vi "solar_cfg Core Edit.vi"(6 "Write Comments? (T)":bool=TRUE, 7 "Action (Read)":enum8{"Read", "Write", "Parse", "Build"}(ring), 8 "error in (no error)":errorcluster, 9 "kvc in":string[](array[string]), 10 "Section/String in":string, 11 "Sections in":cluster{"Section":string, "kvc":string[][]}[](array[cluster])) -> (0 "error out":errorcluster, 1 "Found?":bool, 2 "Value/String out":string, 3 "Sections out":cluster{"Section":string, "kvc":string[][]}[](array[cluster]), 5 "Dirty?":bool)   [LabVIEW 2018]
doc: "This VI parses the configuration string to sections, keys, values and comments."
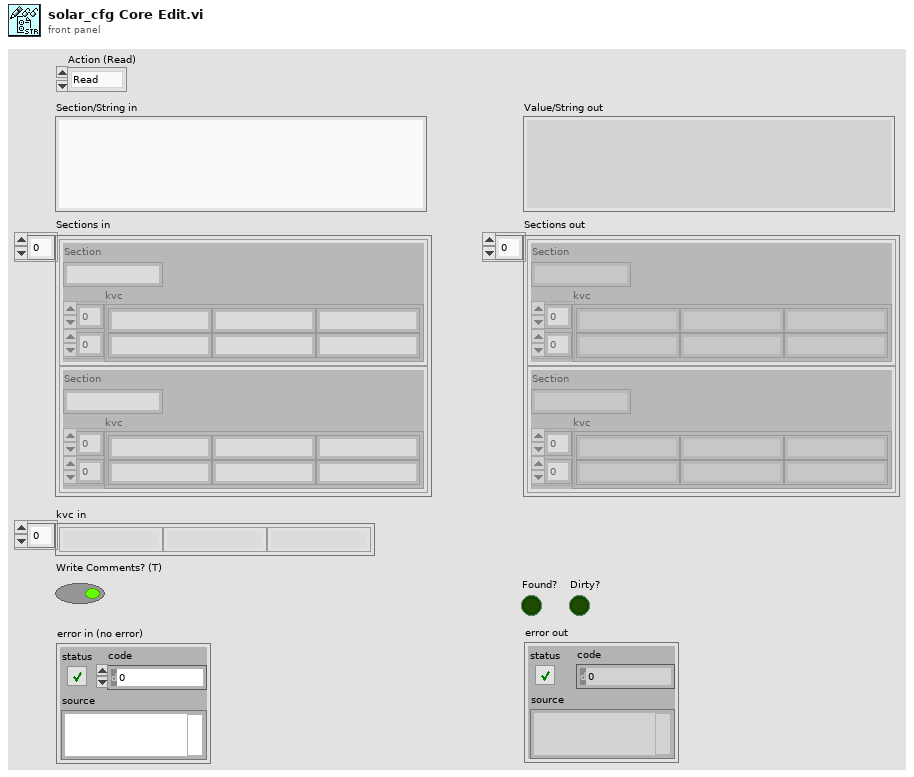
[diagram p1: front panel]
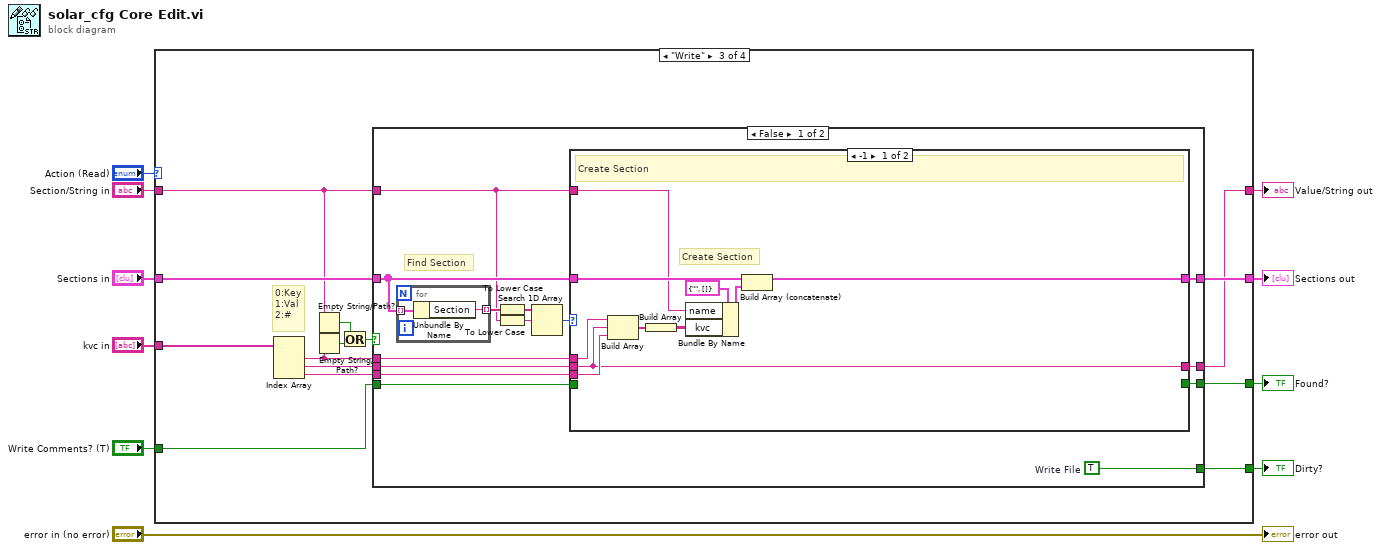
[diagram p0: block diagram]
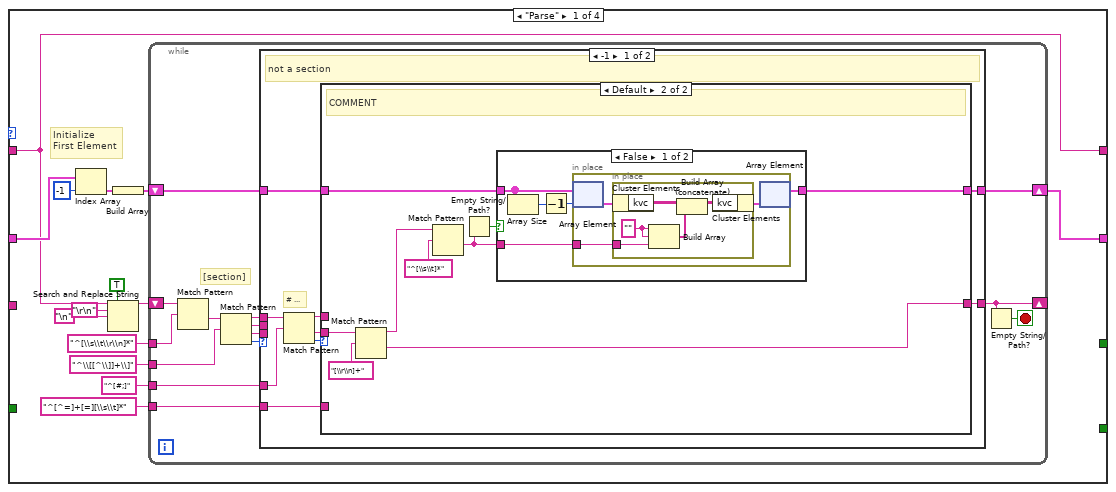
[diagram p2: hidden frame]
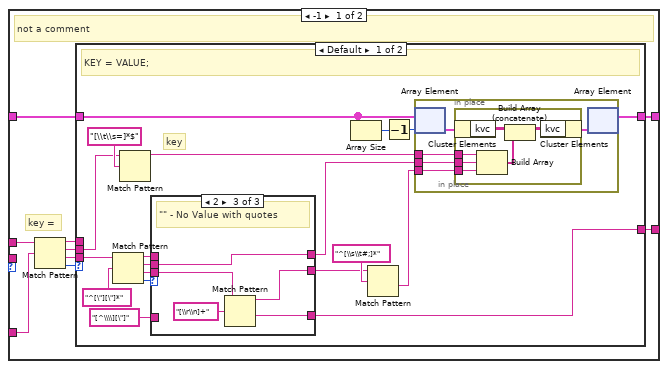
[diagram p3: hidden frame]
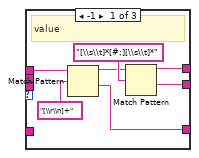
[diagram p4: hidden frame]
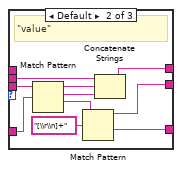
[diagram p5: hidden frame]
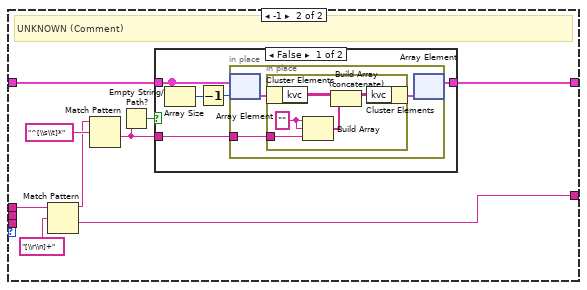
[diagram p6: hidden frame]
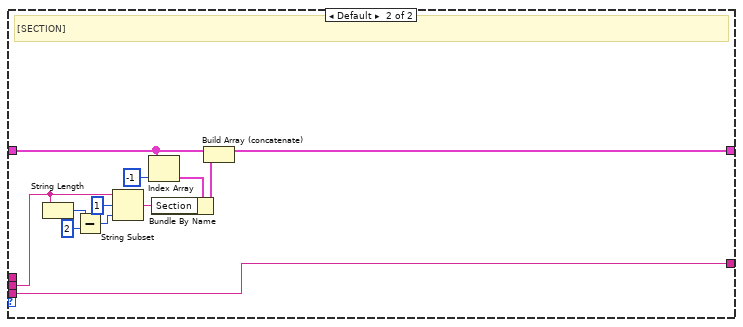
[diagram p9: hidden frame]
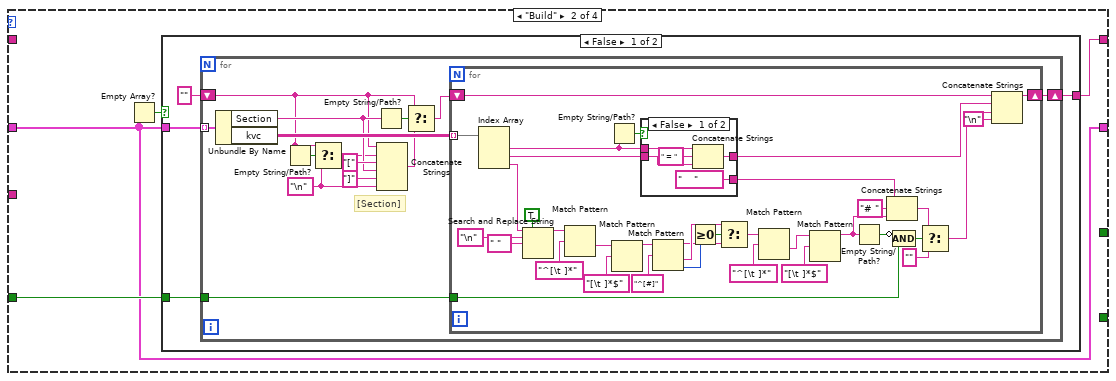
[diagram p10: hidden frame]
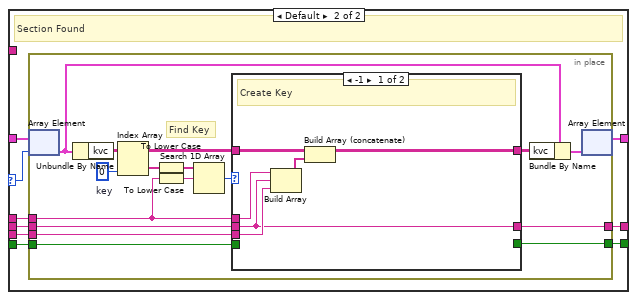
[diagram p13: hidden frame]
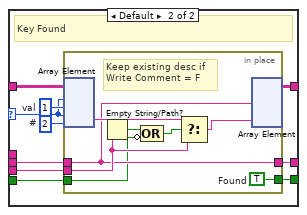
[diagram p14: hidden frame]
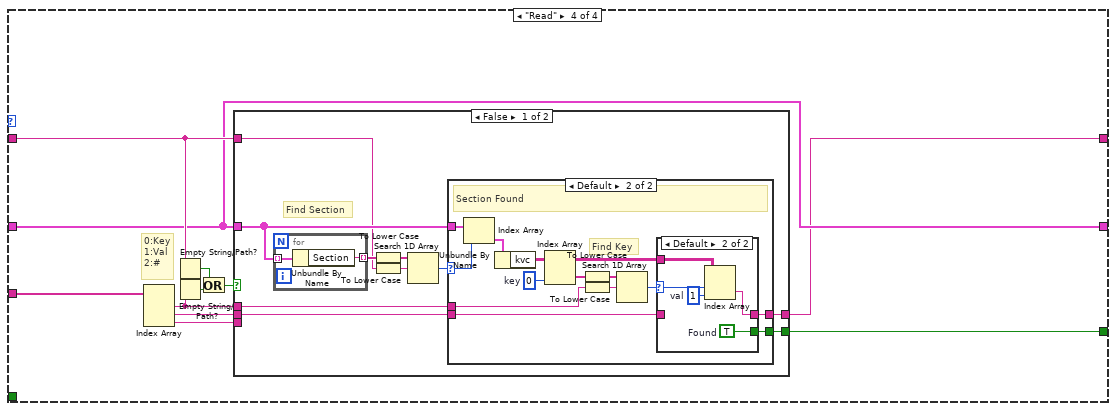
[diagram p16: hidden frame]
diagram:
  n1 = case shown="\"Write\"" "Action (Read)" {
    tunnel: "Section/String in" -> [w12 _ w233 w328]
    tunnel: [w11 w168 w241 w320] -> w9
    tunnel: [w12 w170 w232 w319] -> w7
    tunnel: "Sections in" -> [w13 w168 w242 w320]
    tunnel: "Write Comments? (T)" -> [_ w169 w231 _]
    tunnel: "kvc in" -> [_ _ w240 w329]
    tunnel: [_ _ w239 w327] -> w3
    tunnel: [_ _ w238 _] -> w2
    frame "Parse" {
      # "Initialize\nFirst Element"
      n2 = Index Array(array=w13, index=-1) -> (element=w19:cluster{"Section":string, "kvc":string[][]})
      n3 = Search and Replace String(replace all?=TRUE ("replace all? (F)"), input string=w12, search string="\r\n" ("End of Line Constant"), replace string="\n" ("Line Feed Constant")) -> (result string=w24:string)  [unwired: 4 in, 3 out]
      n4 = Build Array(w19) -> (w18:cluster{"Section":string, "kvc":string[][]}[])
      n5 = while {
        shift-right: [w30] -> _
        shift-left: w24 -> [w38]
        shift-right: [w31] -> w11
        shift-left: w18 -> [w32]
        tunnel: "^[\\s\\t\\r\\n]*" ("regular expression") -> [w28]
        tunnel: "^\\[[^\\]]+\\]" -> [w27]
        tunnel: "^[#;]" -> [w26]
        tunnel: "^[^=]+[=][\\s\\t]*" -> [w25]
        stop <- w29 stop-if-true
        # "[section]"
        n6 = Match Pattern(string=w38, regular expression=w28) -> (after substring=w37:string)  [unwired: 1 in, 3 out]
        n7 = Match Pattern(string=w37, regular expression=w27) -> (before substring=w35:string, match substring=w34:string, after substring=w33:string, offset past match=w36:i32)  [unwired: 1 in]
        n8 = case shown="-1" w36 {
          tunnel: w35 -> [w47 _]
          tunnel: w34 -> [_ w164]
          tunnel: w33 -> [_ w166]
          tunnel: [w42 w166] -> w30
          tunnel: w32 -> [w44 w159]
          tunnel: [w45 w160] -> w31
          tunnel: w26 -> [w40 _]
          tunnel: w25 -> [w39 _]
          frame -1 {
            # "# ..."
            # "not a section"
            n9 = Match Pattern(string=w47, regular expression=w40) -> (before substring=w41:string, after substring=w43:string, offset past match=w46:i32)  [unwired: 1 in, 1 out]
            n10 = case shown="Default" w46 {
              tunnel: [w54 w139] -> w45
              tunnel: w44 -> [w53 w140]
              tunnel: w43 -> [_ w137]
              tunnel: [w49 w136] -> w42
              tunnel: w41 -> [w56 _]
              tunnel: w39 -> [w48 _]
              frame -1 {
                # "key ="
                # "not a comment"
                n11 = Match Pattern(string=w56, regular expression=w48) -> (before substring=w52:string, match substring=w50:string, after substring=w51:string, offset past match=w55:i32)  [unwired: 1 in]
                n12 = case shown="Default" w55 {
                  tunnel: [w72 w116] -> w54
                  tunnel: w53 -> [w73 w117]
                  tunnel: w52 -> [_ w114]
                  tunnel: w51 -> [w67 _]
                  tunnel: w50 -> [w70 _]
                  tunnel: [w58 w113] -> w49
                  frame Default {
                    # "key"
                    # "KEY = VALUE;"
                    n13 = Match Pattern(string=w67, regular expression="^[\"][\"]*") -> (before substring=w57:string, match substring=w61:string, after substring=w64:string, offset past match=w65:i32)  [unwired: 1 in]
                    n14 = Match Pattern(string=w70, regular expression="[\\t\\s=]*$") -> (before substring=w69:string)  [unwired: 1 in, 3 out]
                    n15 = case shown="2" w65 {
                      tunnel: w64 -> [_ w92 w94]
                      tunnel: "[^\\\\][\"]" -> [_ w91 _]
                      tunnel: [w77 w83 w93] -> w62
                      tunnel: w61 -> [_ w86 w93]
                      tunnel: [w76 w88 w96] -> w60
                      tunnel: [w80 w87 w95] -> w58
                      tunnel: w57 -> [w81 _ _]
                      frame -1 {
                        # "value"
                        n16 = Match Pattern(string=w81, regular expression="[\\r\\n]+") -> (before substring=w78:string, after substring=w80:string)  [unwired: 1 in, 2 out]
                        n17 = Match Pattern(string=w78, regular expression="[\\s\\t]*[#;][\\s\\t]*") -> (before substring=w77:string, after substring=w76:string)  [unwired: 1 in, 2 out]
                      }
                      frame Default {
                        # "\"value\""
                        n18 = Match Pattern(string=w92, regular expression=w91) -> (before substring=w85:string, match substring=w84:string, after substring=w89:string)  [unwired: 1 in, 1 out]
                        n19 = Match Pattern(string=w89, regular expression="[\\r\\n]+") -> (before substring=w88:string, after substring=w87:string)  [unwired: 1 in, 2 out]
                        n20 = Concatenate Strings(w86, w85, w84) -> (w83:string)
                      }
                      frame 2 {
                        # "\"\" - No Value with quotes"
                        n21 = Match Pattern(string=w94, regular expression="[\\r\\n]+") -> (before substring=w96:string, after substring=w95:string)  [unwired: 1 in, 2 out]
                      }
                    }
                    n22 = Array Size(array=w73) -> (size(s)=w75:i32)
                    n23 = Match Pattern(string=w60, regular expression="^[\\s\\t#;]*") -> (after substring=w59:string)  [unwired: 1 in, 3 out]
                    n24 = Decrement(x=w75) -> (x-1=w74:i32)
                    n25 = in-place {
                      in-place-border: w59 -> [w101]
                      in-place-border: w69 -> [w99]
                      in-place-border: w62 -> [w98]
                      n26 = in-place-array #1(w73, w74) -> (w102:cluster{"Section":string, "kvc":string[][]})
                      n27 = in-place {
                        in-place-border: w101 -> [w106]
                        in-place-border: w99 -> [w104]
                        in-place-border: w98 -> [w103]
                        n28 = in-place-cluster #2(w102) -> ("kvc"=w108:string[][])
                        n29 = Build Array(w104, w103, w106) -> (w105:string[])
                        n30 = Build Array (concatenate)(w108, w105) -> (w107:string[][])
                        n31 = in-place-cluster #2("kvc"=w107) -> (w100:cluster{"Section":string, "kvc":string[][]})
                      }
                      n32 = in-place-array #1(w100) -> (w72:cluster{"Section":string, "kvc":string[][]}[])  [unwired: 1 out]
                    }
                  }
                  frame -1 {
                    # "UNKNOWN (Comment)"
                    n33 = Match Pattern(string=w114, regular expression="[\\r\\n]+") -> (before substring=w110:string, after substring=w113:string)  [unwired: 1 in, 2 out]
                    n34 = Match Pattern(string=w110, regular expression="^[\\s\\t]*") -> (after substring=w109:string)  [unwired: 1 in, 3 out]
                    n35 = Empty String/Path?(string/path=w109) -> (empty?=w112:bool)
                    n36 = case shown="False" w112 {
                      tunnel: w117 -> [w120 w131]
                      tunnel: [w119 w131] -> w116
                      tunnel: w109 -> [w118 _]
                      frame False {
                        n37 = Array Size(array=w120) -> (size(s)=w122:i32)
                        n38 = Decrement(x=w122) -> (x-1=w121:i32)
                        n39 = in-place {
                          in-place-border: w118 -> [w124]
                          n40 = in-place-array #3(w120, w121) -> (w125:cluster{"Section":string, "kvc":string[][]})
                          n41 = in-place {
                            in-place-border: w124 -> [w127]
                            w128 = ""
                            n42 = in-place-cluster #4(w125) -> ("kvc"=w130:string[][])
                            n43 = Build Array(w128, w128, w127) -> (w126:string[])
                            n44 = Build Array (concatenate)(w130, w126) -> (w129:string[][])
                            n45 = in-place-cluster #4("kvc"=w129) -> (w123:cluster{"Section":string, "kvc":string[][]})
                          }
                          n46 = in-place-array #3(w123) -> (w119:cluster{"Section":string, "kvc":string[][]}[])  [unwired: 1 out]
                        }
                      }
                      frame True {
                      }
                    }
                  }
                }
              }
              frame Default {
                # "COMMENT"
                n47 = Match Pattern(string=w137, regular expression="[\\r\\n]+") -> (before substring=w132:string, after substring=w136:string)  [unwired: 1 in, 2 out]
                n48 = Match Pattern(string=w132, regular expression="^[\\s\\t]*") -> (after substring=w133:string)  [unwired: 1 in, 3 out]
                n49 = Empty String/Path?(string/path=w133) -> (empty?=w135:bool)
                n50 = case shown="False" w135 {
                  tunnel: w140 -> [w145 w154]
                  tunnel: [w142 w154] -> w139
                  tunnel: w133 -> [w141 _]
                  frame False {
                    n51 = Array Size(array=w145) -> (size(s)=w144:i32)
                    n52 = Decrement(x=w144) -> (x-1=w143:i32)
                    n53 = in-place {
                      in-place-border: w141 -> [w147]
                      n54 = in-place-array #5(w145, w143) -> (w148:cluster{"Section":string, "kvc":string[][]})
                      n55 = in-place {
                        in-place-border: w147 -> [w150]
                        w151 = ""
                        n56 = in-place-cluster #6(w148) -> ("kvc"=w153:string[][])
                        n57 = Build Array(w151, w151, w150) -> (w149:string[])
                        n58 = Build Array (concatenate)(w153, w149) -> (w152:string[][])
                        n59 = in-place-cluster #6("kvc"=w152) -> (w146:cluster{"Section":string, "kvc":string[][]})
                      }
                      n60 = in-place-array #5(w146) -> (w142:cluster{"Section":string, "kvc":string[][]}[])  [unwired: 1 out]
                    }
                  }
                  frame True {
                  }
                }
              }
            }
          }
          frame Default {
            # "[SECTION]"
            n61 = String Length(string=w164) -> (length=w163:i32)
            n62 = Subtract(x=w163, y=2) -> (x-y=w162:i32)
            n63 = String Subset(string=w164, offset (0)=1, length (rest)=w162) -> (substring=w156:string)
            n64 = Index Array(array=w159, index=-1) -> (element=w157:cluster{"Section":string, "kvc":string[][]})
            n65 = Bundle By Name(cluster=w157, "Section"=w156) -> (w155:cluster{"Section":string, "kvc":string[][]})
            n66 = Build Array (concatenate)(w159, w155) -> (w160:cluster{"Section":string, "kvc":string[][]}[])
          }
        }
        n67 = Empty String/Path?(string/path=w30) -> (empty?=w29:bool)
      }
    }
    frame "Build" {
      n68 = Empty Array?(array=w168) -> (empty?=w167:bool)
      n69 = case shown="False" w167 {
        tunnel: w168 -> [w173 _]
        tunnel: [w172 _] -> w170
        tunnel: w169 -> [w171 _]
        frame False {
          n70 = for {
            tunnel: w173 -> [w188] mode=indexing
            shift-right: [w187] -> w172
            shift-left: "" -> [w177]
            tunnel: w171 -> [w186]
            w175 = "\n" ("string")
            # "[Section]"
            n71 = Unbundle By Name(w188) -> ("Section"=w180:string, "kvc"=w185:string[][])
            n72 = Empty String/Path?(string/path=w177) -> (empty?=w178:bool)
            n73 = Select(t=w177, s=w178, f=w175) -> (s? t:f=w176:string)
            n74 = Empty String/Path?(string/path=w180) -> (empty?=w184:bool)
            n75 = Concatenate Strings(w177, w176, "[" ("string"), w180, "]" ("string"), w175) -> (w183:string)
            n76 = Select(t=w177, s=w184, f=w183) -> (s? t:f=w179:string)
            n77 = for {
              tunnel: w186 -> [w201]
              tunnel: w185 -> [w195] mode=indexing
              shift-right: [w221] -> w187
              shift-left: w179 -> [w218]
              n78 = Index Array(array=w195) -> (element #1=w220:string, element #2=w219:string, element #3=w215:string)  [unwired: 3 in]
              n79 = Search and Replace String(replace all?=TRUE ("replace all? (F)"), input string=w215, search string="\n", replace string=" " ("replace string (\"\")")) -> (result string=w214:string)  [unwired: 4 in, 3 out]
              n80 = Match Pattern(string=w214, regular expression="^[\t ]*") -> (after substring=w212:string)  [unwired: 1 in, 3 out]
              n81 = Empty String/Path?(string/path=w220) -> (empty?=w194:bool)
              n82 = Match Pattern(string=w212, regular expression="[\t ]*$") -> (before substring=w210:string)  [unwired: 1 in, 3 out]
              n83 = case shown="False" w194 {
                tunnel: w220 -> [w228 _]
                tunnel: w219 -> [w226 _]
                tunnel: [w225 _] -> w223
                tunnel: ["    " ("string") _] -> w196
                frame False {
                  n84 = Concatenate Strings(w228, " = " ("string"), w226) -> (w225:string)
                }
                frame True {
                }
              }
              n85 = Match Pattern(string=w210, regular expression="^[#]" ("string")) -> (before substring=w203:string, after substring=w204:string, offset past match=w206:i32)  [unwired: 1 in, 1 out]
              n86 = Greater Or Equal To 0?(x=w206) -> (x >= 0?=w205:bool)
              n87 = Select(t=w204, s=w205, f=w203) -> (s? t:f=w190:string)
              n88 = Match Pattern(string=w190, regular expression="^[\t ]*") -> (after substring=w193:string)  [unwired: 1 in, 3 out]
              n89 = Match Pattern(string=w193, regular expression="[\t ]*$") -> (before substring=w189:string)  [unwired: 1 in, 3 out]
              n90 = Empty String/Path?(string/path=w189) -> (empty?=w202:bool)
              n91 = Concatenate Strings(w196, "# " ("string"), w189) -> (w208:string)
              n92 = Compound Arithmetic op=AND(invert w202, w201) -> (w200:bool)
              n93 = Select(t=w208, s=w200, f="") -> (s? t:f=w207:string)
              n94 = Concatenate Strings(w218, w223, w207, "\n" ("Line Feed Constant")) -> (w221:string)
            }
          }
        }
        frame True {
        }
      }
    }
    frame "Write" {
      # "0:Key\n1:Val\n2:#"
      n95 = Index Array(array=w240) -> (element #1=w234:string, element #2=w235:string, element #3=w230:string)  [unwired: 3 in]
      n96 = Empty String/Path?(string/path=w233) -> (empty?=w237:bool)
      n97 = Empty String/Path?(string/path=w234) -> (empty?=w229:bool)
      n98 = Or(x=w237, y=w229) -> (x .or. y?=w236:bool)
      n99 = case "Section or Key Empty?" shown="False" w236 {
        tunnel: [w256 _] -> w239
        tunnel: [w244 w317] -> w232
        tunnel: w242 -> [w247 w318]
        tunnel: [w255 _] -> w238
        tunnel: [w254 w318] -> w241
        tunnel: w235 -> [w252 w317]
        tunnel: w233 -> [w246 _]
        tunnel: w230 -> [w251 _]
        tunnel: w234 -> [w253 _]
        tunnel: w231 -> [w243 _]
        frame False {
          w255 = TRUE  # Write File
          # "Find Section"
          # "Section & Key Valid"
          n100 = for {
            tunnel: w247 -> [w316] mode=indexing
            tunnel: [w315] -> w250 mode=indexing
            n101 = Unbundle By Name(w316) -> ("Section"=w315:string)
          }
          n102 = To Lower Case(string=w250) -> (all lower case string=w249:string[])
          n103 = To Lower Case(string=w246) -> (all lower case string=w248:string)
          n104 = Search 1D Array(1D array=w249, element=w248) -> (index of element=w245:i32)  [unwired: 1 in]
          n105 = case "Section Exists?" shown="-1" w245 {
            selector: w245 -> [_ w268]
            tunnel: w247 -> [w266 w271]
            tunnel: w253 -> [w264 w275]
            tunnel: w246 -> [w257 _]
            tunnel: [_ w274] -> w256
            tunnel: w252 -> [w258 w273]
            tunnel: [w258 w272] -> w244
            tunnel: [w265 w270] -> w254
            tunnel: w251 -> [w263 w269]
            tunnel: w243 -> [_ w267]
            frame -1 {
              # "Create Section"
              # "Create Section"
              n106 = Build Array(w264, w258, w263) -> (w260:string[])
              n107 = Build Array(w260) -> (w259:string[][])
              n108 = Bundle By Name(cluster=cluster{"name":string, "kvc":string[][]} {"name"="", "kvc"=[]} ("Section"), "name"=w257, "kvc"=w259) -> (w261:cluster{"name":string, "kvc":string[][]})
              n109 = Build Array (concatenate)(w266, w261) -> (w265:cluster{"name":string, "kvc":string[][]}[])
            }
            frame Default {
              # "Section Found"
              n110 = in-place {
                in-place-border: w275 -> [w290]
                in-place-border: [w289] -> w274
                in-place-border: w273 -> [w288]
                in-place-border: [w287] -> w272
                in-place-border: w269 -> [w284]
                in-place-border: w267 -> [w276]
                w283 = 0  # key
                # "Find Key"
                n111 = in-place-array #7(w271, w268) -> (w286:cluster{"Section":string, "kvc":string[][]})
                n112 = Unbundle By Name(w286) -> ("kvc"=w280:string[][])
                n113 = Index Array(array=w280, index (col)=w283) -> (element=w278:string[])  [unwired: 1 in]
                n114 = To Lower Case(string=w278) -> (all lower case string=w282:string[])
                n115 = To Lower Case(string=w290) -> (all lower case string=w281:string)
                n116 = Search 1D Array(1D array=w282, element=w281) -> (index of element=w277:i32)  [unwired: 1 in]
                n117 = case "Key Exists?" shown="-1" w277 {
                  selector: w277 -> [_ w299]
                  tunnel: w290 -> [w294 _]
                  tunnel: w280 -> [w296 w306]
                  tunnel: [_ w298] -> w289
                  tunnel: w288 -> [w291 w303]
                  tunnel: [w291 w305] -> w287
                  tunnel: [w295 w304] -> w279
                  tunnel: w284 -> [w293 w302]
                  tunnel: w276 -> [_ w297]
                  frame -1 {
                    # "Create Key"
                    n118 = Build Array(w294, w291, w293) -> (w292:string[])
                    n119 = Build Array (concatenate)(w296, w292) -> (w295:string[][])
                  }
                  frame Default {
                    w300 = 2  # #
                    w301 = 1  # val
                    # "Key Found"
                    n120 = in-place {
                      in-place-border: w303 -> [w310]
                      in-place-border: [w310] -> w305
                      in-place-border: w302 -> [w313]
                      in-place-border: [w311] -> w298
                      in-place-border: w297 -> [w309]
                      w311 = TRUE  # Found
                      # "Keep existing desc if \nWrite Comment = F"
                      n121 = in-place-array #8(w306, w299, w301, w299, w300) -> (w314:string)  [unwired: 1 out]
                      n122 = Empty String/Path?(string/path=w313) -> (empty?=w308:bool)
                      n123 = Compound Arithmetic op=OR(w308, invert w309) -> (w307:bool)
                      n124 = Select(t=w314, s=w307, f=w313) -> (s? t:f=w312:string)
                      n125 = in-place-array #8(w310, w312) -> (w304:string[][])  [unwired: 4 out]
                    }
                  }
                }
                n126 = Bundle By Name(cluster=w286, "kvc"=w279) -> (w285:cluster{"Section":string, "kvc":string[][]})
                n127 = in-place-array #7(w285) -> (w270:cluster{"Section":string, "kvc":string[][]}[])  [unwired: 1 out]
              }
            }
          }
        }
        frame True {
          # "Invalid Section & Key - Do Nothing"
        }
      }
    }
    frame "Read" {
      # "0:Key\n1:Val\n2:#"
      n128 = Index Array(array=w329) -> (element #1=w321:string, element #2=w323:string, element #3=w322:string)  [unwired: 3 in]
      n129 = Empty String/Path?(string/path=w328) -> (empty?=w325:bool)
      n130 = Empty String/Path?(string/path=w321) -> (empty?=w326:bool)
      n131 = Or(x=w325, y=w326) -> (x .or. y?=w324:bool)
      n132 = case "Section or Key Empty?" shown="False" w324 {
        tunnel: [w339 _] -> w327
        tunnel: [w338 w362] -> w319
        tunnel: w320 -> [w332 _]
        tunnel: w323 -> [w336 w362]
        tunnel: w328 -> [w330 _]
        tunnel: w322 -> [_ _]
        tunnel: w321 -> [w337 _]
        frame False {
          # "Find Section"
          # "Section & Key Valid"
          n133 = for {
            tunnel: w332 -> [w361] mode=indexing
            tunnel: [w360] -> w335 mode=indexing
            n134 = Unbundle By Name(w361) -> ("Section"=w360:string)
          }
          n135 = To Lower Case(string=w335) -> (all lower case string=w334:string[])
          n136 = To Lower Case(string=w330) -> (all lower case string=w333:string)
          n137 = Search 1D Array(1D array=w334, element=w333) -> (index of element=w331:i32)  [unwired: 1 in]
          n138 = case "Section Exists?" shown="Default" w331 {
            selector: w331 -> [_ w349]
            tunnel: w332 -> [_ w341]
            tunnel: w337 -> [_ w353]
            tunnel: [_ w352] -> w339
            tunnel: w336 -> [w340 w351]
            tunnel: [w340 w350] -> w338
            frame -1 {
              # "Section Not Found"
            }
            frame Default {
              w348 = 0  # key
              # "Find Key"
              # "Section Found"
              n139 = Index Array(array=w341, index=w349) -> (element=w342:cluster{"Section":string, "kvc":string[][]})
              n140 = Unbundle By Name(w342) -> ("kvc"=w345:string[][])
              n141 = Index Array(array=w345, index (col)=w348) -> (element=w344:string[])  [unwired: 1 in]
              n142 = To Lower Case(string=w344) -> (all lower case string=w347:string[])
              n143 = To Lower Case(string=w353) -> (all lower case string=w346:string)
              n144 = Search 1D Array(1D array=w347, element=w346) -> (index of element=w343:i32)  [unwired: 1 in]
              n145 = case "Key Exists?" shown="Default" w343 {
                selector: w343 -> [_ w358]
                tunnel: w345 -> [_ w356]
                tunnel: [_ w357] -> w352
                tunnel: w351 -> [w354 _]
                tunnel: [w354 w355] -> w350
                frame -1 {
                  # "Key Not Found"
                }
                frame Default {
                  w357 = TRUE  # Found
                  w359 = 1  # val
                  # "Key Found"
                  n146 = Index Array(array=w356, index (row)=w358, index (col)=w359) -> (element=w355:string)
                }
              }
            }
          }
        }
        frame True {
          # "Invalid Section & Key - Do Nothing"
        }
      }
    }
  }
  "Sections out" <- w9
  "Value/String out" <- w7
  "Found?" <- w3
  "Dirty?" <- w2
  "error out" <- "error in (no error)"
